vi "Global Benchmark Call.vi"(8 "error in":errorcluster, 10 "Count":i32=10000, 11 "Log Instance":refnum<class "LoggerReference.lvclass">) -> (0 "error out":errorcluster, 3 "Call Times":dbl[](array[numeric]))   [LabVIEW 2017, in "Benchmarking.lvclass"]
uses:
  Benchmarking.lvclass
  Source/Composed Log/LoggerReference/LoggerReference.lvclass
  Source/Composed Log/Types/Log Level.ctl
  Source/Composed Log/LoggerReference/LoggerReference.lvclass/LoggerReference.ctl
  Source/Composed Log/LoggerReference/Log.vi
  Source/Composed Log/LoggerReference/Remove Stale Logs.vi
  Source/Composed Log/Singleton Event Log/Logger Queue FGV.vi
  Source/Composed Log/Composed Log.lvlib
  Source/Composed Log/Singleton Event Log/Singleton Event Log.lvlib
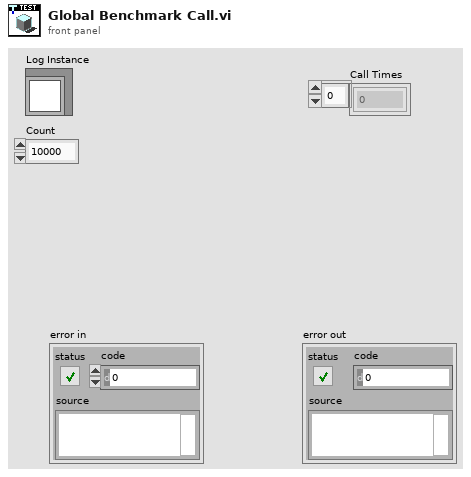
[diagram p1: front panel]
types:
  T1 = typedef "Composed Log.lvlib/Log Level.ctl" = enum16{"Debug", "Info", "Warning", "Error", "Critical"}
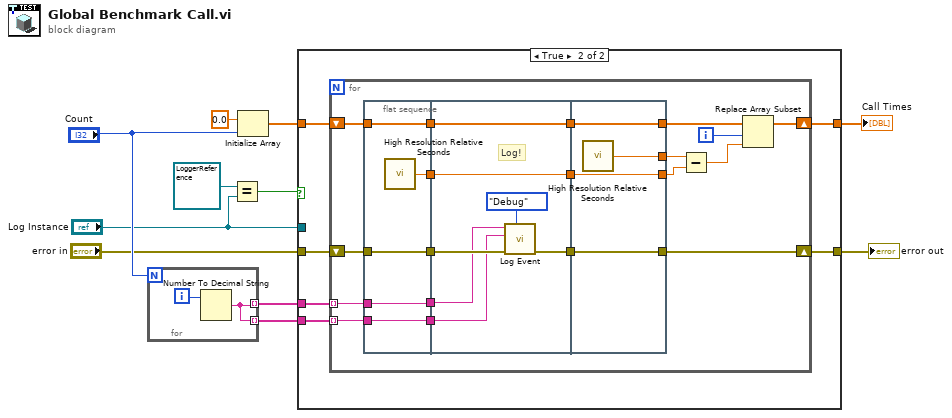
[diagram p0: block diagram]
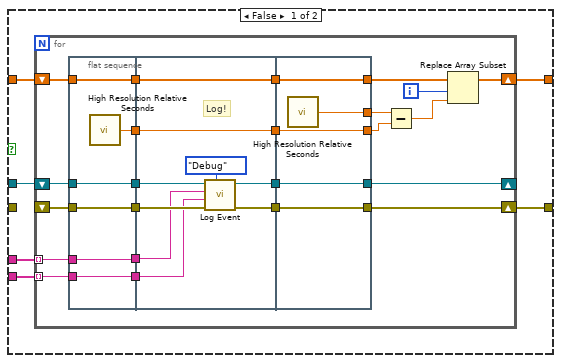
[diagram p2: hidden frame]
diagram:
  n1 = for {
    N: "Count" -> [_]
    tunnel: [w12] -> w7 mode=indexing
    tunnel: [w12] -> w6 mode=indexing
    i -> [w13]
    n2 = Number To Decimal String(number=w13) -> (decimal integer string=w12:string)  [unwired: 1 in]
  }
  n3 = Equal?(x=refnum<class "LoggerReference.lvclass"> refnum, y="Log Instance") -> (x = y?=w1:bool)
  n4 = Initialize Array(0.0 ("element"), "Count") -> (w10:dbl[])
  n5 = case shown="True" w1 {
    tunnel: w10 -> [w17 w68]
    tunnel: "error in" -> [_ w67]
    tunnel: w7 -> [w19 w66]
    tunnel: w6 -> [w18 w65]
    tunnel: [w15 w64] -> w5
    tunnel: [w16 w63] -> w4
    tunnel: "Log Instance" -> [w14 _]
    frame False {
      n6 = for {
        tunnel: w19 -> [w37] mode=indexing
        shift-right: [w35] -> w15
        shift-left: _ -> [w36]
        shift-right: [w26] -> w16
        shift-left: w17 -> [w32]
        tunnel: w18 -> [w25] mode=indexing
        shift-right: [w20] -> _
        shift-left: w14 -> [w23]
        i -> [w28]
        n7 = flat-sequence {
          tunnel: w36 -> [w47]
          tunnel: w37 -> [w48]
          tunnel: [w48] -> w42
          tunnel: [w47] -> w41
          tunnel: [w46] -> w40
          tunnel: w32 -> [w45]
          tunnel: [w45] -> w30
          tunnel: w25 -> [w44]
          tunnel: [w44] -> w24
          tunnel: w23 -> [w43]
          tunnel: [w43] -> w22
          tunnel: w42 -> [w52]
          tunnel: w41 -> [w56]
          tunnel: w40 -> [w54]
          tunnel: [w55] -> w39
          tunnel: [w54] -> w38
          tunnel: [w53] -> w31
          tunnel: w30 -> [w53]
          tunnel: w24 -> [w51]
          tunnel: w22 -> [w50]
          tunnel: [w49] -> w21
          tunnel: [w61] -> w34
          tunnel: [w62] -> w35
          tunnel: w39 -> [w62]
          tunnel: w38 -> [w61]
          tunnel: [w60] -> w33
          tunnel: [w59] -> w29
          tunnel: w31 -> [w59]
          tunnel: w21 -> [w58]
          tunnel: [w58] -> w20
          frame #0 {
            n8 = call <vilib>:"High Resolution Relative Seconds.vi"() -> ("relative seconds"=w46:dbl)
          }
          frame #1 {
            # "Log!"
            n9 = call "Log Event.vi"("Event Level"=Log_Level."Debug", "error in (no error)"=w56, "Data To Log"=w51, "SourceID"=w52, "Log Instance"=w50) -> ("error out"=w55:errorcluster, "Log Instance Out"=w49:refnum<class "LoggerReference.lvclass">)  [unwired: 5 in]
          }
          frame #2 {
            n10 = call <vilib>:"High Resolution Relative Seconds.vi"() -> ("relative seconds"=w60:dbl)
          }
        }
        n11 = Subtract(x=w33, y=w34) -> (x-y=w27:dbl)
        n12 = Replace Array Subset(array=w29, new element=w27, index=w28) -> (w26:dbl[])
      }
    }
    frame True {
      n13 = for {
        tunnel: w66 -> [w82] mode=indexing
        shift-right: [w80] -> w64
        shift-left: w67 -> [w81]
        shift-right: [w71] -> w63
        shift-left: w68 -> [w77]
        tunnel: w65 -> [w70] mode=indexing
        i -> [w73]
        n14 = flat-sequence {
          tunnel: w81 -> [w91]
          tunnel: w82 -> [w92]
          tunnel: [w92] -> w87
          tunnel: [w91] -> w86
          tunnel: [w90] -> w85
          tunnel: w77 -> [w89]
          tunnel: [w89] -> w75
          tunnel: w70 -> [w88]
          tunnel: [w88] -> w69
          tunnel: w87 -> [w95]
          tunnel: w86 -> [w97]
          tunnel: w85 -> [w99]
          tunnel: [w94] -> w84
          tunnel: [w99] -> w83
          tunnel: [w98] -> w76
          tunnel: w75 -> [w98]
          tunnel: w69 -> [w96]
          tunnel: [w102] -> w79
          tunnel: [w103] -> w80
          tunnel: w84 -> [w103]
          tunnel: w83 -> [w102]
          tunnel: [w101] -> w78
          tunnel: [w100] -> w74
          tunnel: w76 -> [w100]
          frame #0 {
            n15 = call <vilib>:"High Resolution Relative Seconds.vi"() -> ("relative seconds"=w90:dbl)
          }
          frame #1 {
            # "Log!"
            n16 = call "Log Event.vi"("Event Level"=Log_Level."Debug", "error in (no error)"=w97, "Data To Log"=w96, "SourceID"=w95) -> ("error out"=w94:errorcluster)  [unwired: 7 in]
          }
          frame #2 {
            n17 = call <vilib>:"High Resolution Relative Seconds.vi"() -> ("relative seconds"=w101:dbl)
          }
        }
        n18 = Subtract(x=w78, y=w79) -> (x-y=w72:dbl)
        n19 = Replace Array Subset(array=w74, new element=w72, index=w73) -> (w71:dbl[])
      }
    }
  }
  "error out" <- w5
  "Call Times" <- w4
